vi "RSNRPZ Set Correction Frequency.vi"(8 "error in (no error)":errorcluster, 9 "Frequency ( 50.0e6 Hz)":dbl=50000000.0 format="%.2p", 10 "Channel (1)":i32=1, 11 "VISA session":refnum<visa-resource-name>) -> (0 "error out":errorcluster, 3 "dup VISA session":refnum<visa-resource-name>)   [LabVIEW 2014]
doc: "This VI informs the R&S NRP about the frequency of the power to be measured since this frequency is not automatically determined. The frequency is used to determine a frequency-dependent correction factor for the measurement results.\n\nRemote-control command(s):\nSENS:FREQ"
uses:
  rsnrpz_32.dll
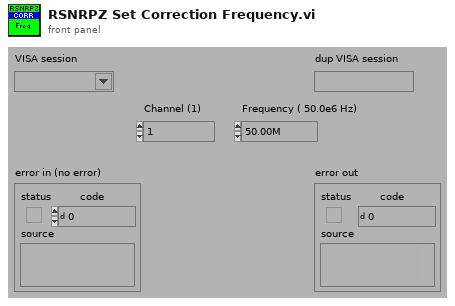
[diagram p1: front panel]
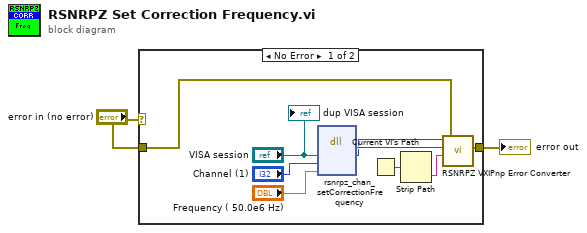
[diagram p0: block diagram]
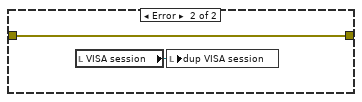
[diagram p2: hidden frame]
diagram:
  n1 = case shown="No Error" "error in (no error)" {
    tunnel: "error in (no error)" -> [w5 w13]
    tunnel: [w6 w13] -> w1
    frame No Error {
      n2 = dll-call lib="rsnrpz_32.dll" fn="rsnrpz_chan_setCorrectionFrequency"("VISA Session"="VISA session", "Channel"="Channel (1)", "Frequency"="Frequency ( 50.0e6 Hz)") -> ("Status"=w10:i32, "VISA Session"=w7:u32)  [unwired: 5 in, 2 out]
      n3 = Current VI's Path() -> (path=w4:path)
      n4 = Strip Path(path=w4) -> (name=w3:string)  [unwired: 1 out]
      n5 = call "RSNRPZ VXIPnp Error Converter.vi"("error in (no error)"=w5, "name of VI"=w3, "VXIPnp error code"=w10, "VISA session"=w7) -> ("error out"=w6:errorcluster)  [unwired: 1 out]
      "dup VISA session" <- "VISA session"
    }
    frame Error {
      n6 = local read "VISA session"() -> (w12:refnum<visa-resource-name>)
      n7 = local write "dup VISA session"(w12) -> ()
    }
  }
  "error out" <- w1
